vi "Main.vi"(11 "Module Admin":refnum<class "Delacor_lib_QMH_Module Admin.lvclass">) -> ()   [LabVIEW 2020, in "Hardware.lvlib"]
doc: "This template is based off of the Queued Message Handler design pattern and the Queued Message Handler project template that ships with LabVIEW.\n\nThe main difference is that the queue is private to this module and communication between modules is performed via Broadcast and Request events.\n\nRequest events are wrapped in public API methods and are handled in the Event Handling Loop (EHL) of this VI. Any module can register for Broadcast events sent by this module. The EHL generates messages based on user interface actions.\n\nThe Message Handling Loop (MHL) processes messages generated by the EHL, or by other messages. The messages are string values, so new messages can be added easily to the Message Cases case structure in the MHL. Each message cluster can also provide an optional value for Message Data, which is a variant that can be converted to whatever message-specific data is required.\n_____\nBased on DQMH Project Template 6.0.0.91."
uses:
  Hardware.lvlib
  <vilib>/Delacor/Delacor QMH/Libraries/Module Admin_class/Delacor_lib_QMH_Module Admin.lvclass
  Module Data--cluster.ctl
  Stop Argument--cluster.ctl
  <vilib>/Delacor/Delacor QMH/Libraries/Message Queue_class/Delacor_lib_QMH_Message Queue.lvclass/Delacor_lib_QMH_Message Queue.ctl
  <vilib>/Delacor/Delacor QMH/Libraries/Module Admin_class/Delacor_lib_QMH_Module Admin.lvclass/Delacor_lib_QMH_Module Admin.ctl
  <vilib>/Utility/miscctls.llb/LVPointTypeDef.ctl
  <vilib>/Delacor/Delacor QMH/Libraries/Message Queue_class/Delacor_lib_QMH_Enqueue Message (Single).vi
  <vilib>/Delacor/Delacor QMH/Libraries/Module Admin_class/Delacor_lib_QMH_Get External Launch.vi
  <vilib>/Utility/error.llb/Error Cluster From Error Code.vi
  <vilib>/ErrorRing/Error Ring.xnode
  <vilib>/Delacor/Delacor QMH/Libraries/Message Queue_class/Delacor_lib_QMH_Message Queue.lvclass
  Paquetes Disponibles/Paquetes Disponibles.lvlib
  Manejador Turnos/Manejador Turnos.lvlib
panel:
  out "error out":errorcluster
  out "Status":string
types:
  T1 = typedef "Hardware.lvlib/Request Events--cluster.ctl" = cluster{"Stop Module":refnum<user-event>, "Show Panel":refnum<user-event>, "Hide Panel":refnum<user-event>, "Get Module Execution Status":refnum<user-event>, "Show Diagram":refnum<user-event>}
  T2 = typedef "Manejador Turnos.lvlib/Broadcast Events--cluster.ctl" = cluster{"Module Did Init":refnum<user-event>, "Status Updated":refnum<user-event>, "Error Reported":refnum<user-event>, "Module Did Stop":refnum<user-event>, "Update Module Execution Status":refnum<user-event>, "Servicio en curso":refnum<user-event>}
  T3 = typedef "Hardware.lvlib/Module Data--cluster.ctl" = cluster{"Status":string, "Servicio":string}
  T4 = enum32{"invalid lock state", "Not Locked", "Locked (No Password)", "Password-protected"}
  T5 = typedef "Hardware.lvlib/Stop Argument--cluster.ctl" = cluster{"Origin":string, "Exit via Stop Module Req?":bool, "Wait for Module to stop?":bool}
  T6 = typedef "LVPointTypeDef.ctl" = cluster{"Horizontal":i16, "Vertical":i16}
  T7 = enum32{"Invalid", "Standard", "Closed", "Hidden", "Minimized", "Maximized"}
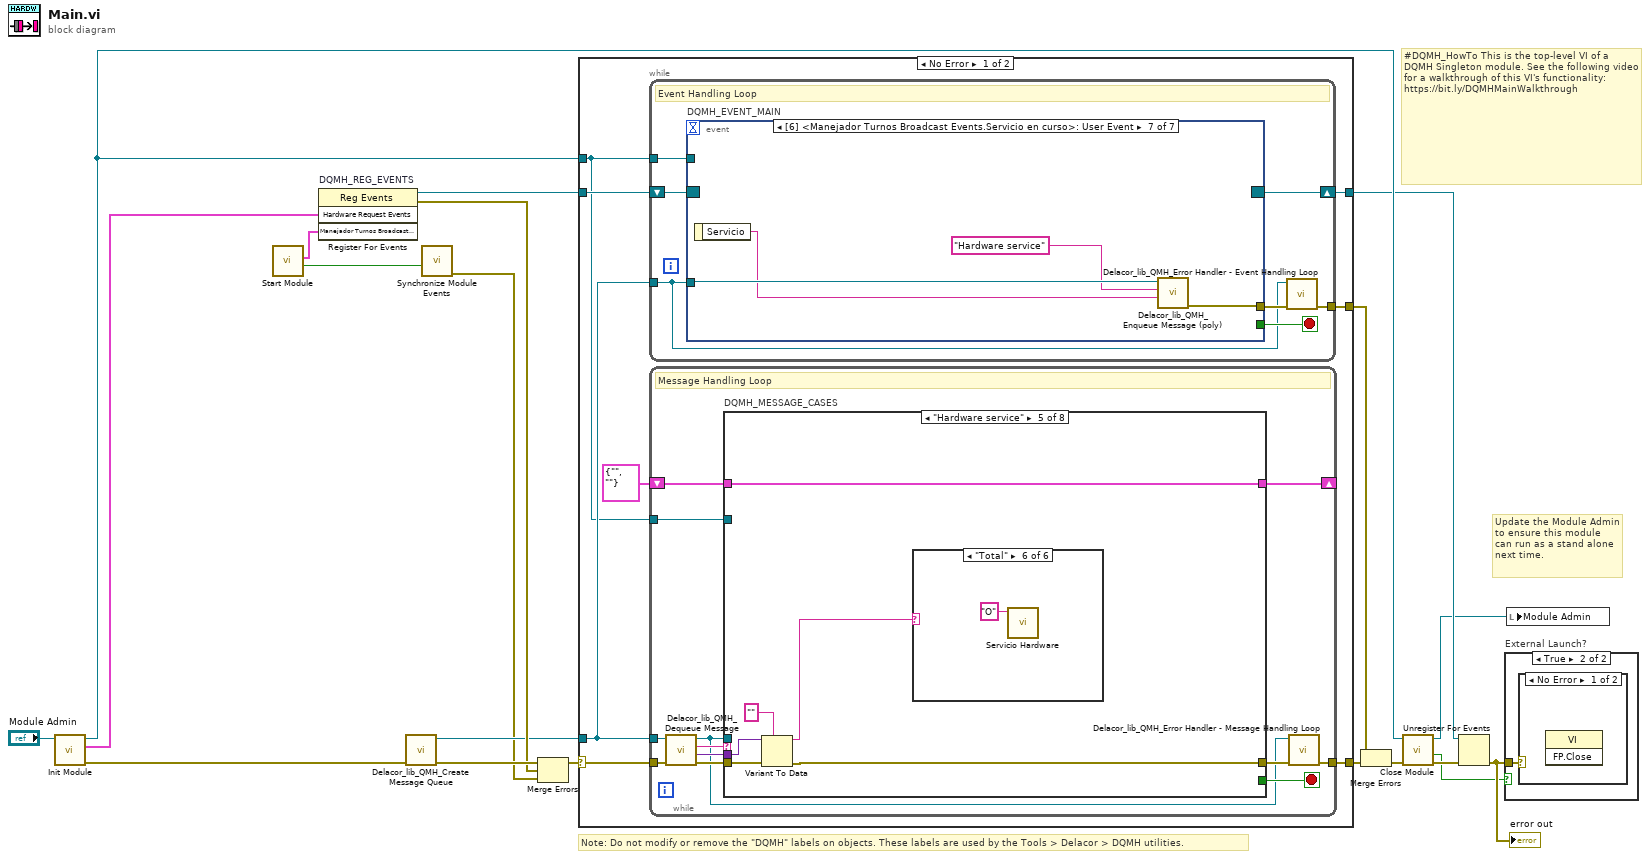
[diagram p0: block diagram]
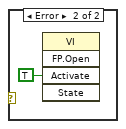
[diagram p3: hidden frame]
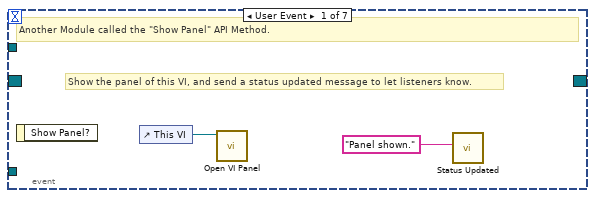
[diagram p4: hidden frame]
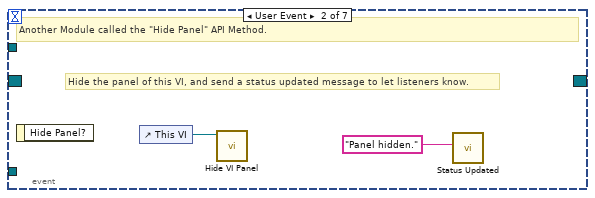
[diagram p5: hidden frame]
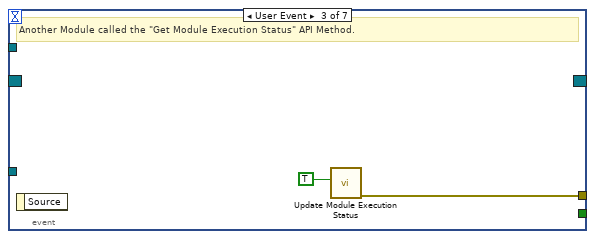
[diagram p6: hidden frame]
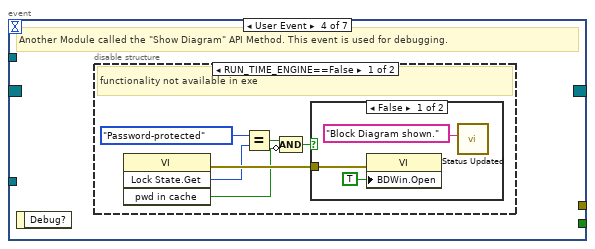
[diagram p7: hidden frame]
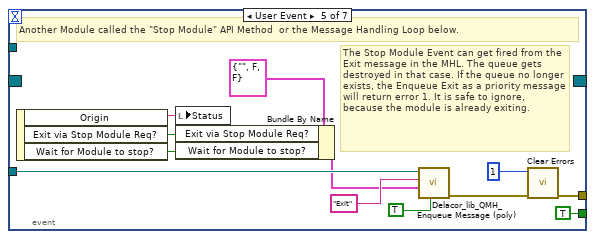
[diagram p10: hidden frame]
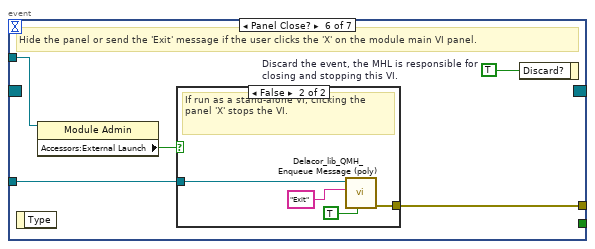
[diagram p11: hidden frame]
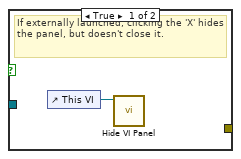
[diagram p12: hidden frame]
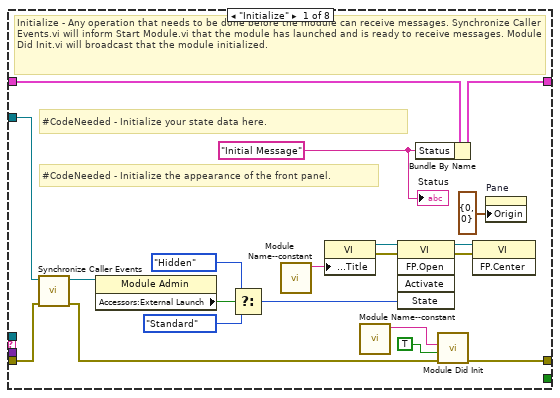
[diagram p13: hidden frame]
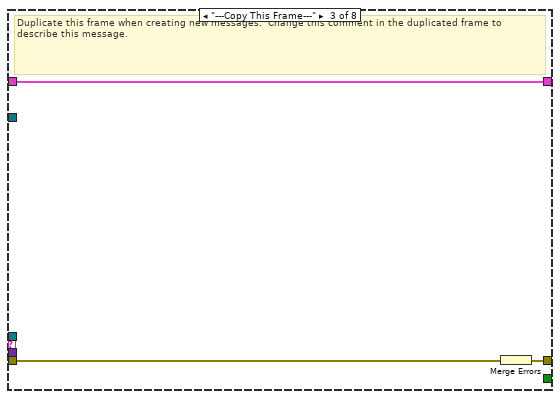
[diagram p15: hidden frame]
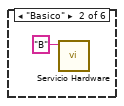
[diagram p18: hidden frame]
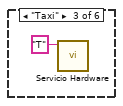
[diagram p19: hidden frame]
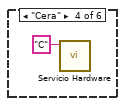
[diagram p20: hidden frame]
diagram:
  # "#DQMH_HowTo This is the top-level VI of a DQMH Singleton module. See the following video for a walkthrough of this VI's functionality: https://bit.ly/DQMHMainWalkthrough"
  # "Note: Do not modify or remove the \"DQMH\" labels on objects. These labels are used by the Tools > Delacor > DQMH utilities."
  # "Update the Module Admin to ensure this module can run as a stand alone next time."
  n1 = call "Init Module.vi"("Singleton Module Admin in"="Module Admin") -> ("error out"=w19:errorcluster, "Hardware Request Events"=w8:T1, "Singleton Module Admin out"=w11:refnum<class "Delacor_lib_QMH_Module Admin.lvclass">)  [unwired: 8 in]
  n2 = call "Start Module.vi"() -> ("Wait for Event Sync?"=w3:bool, "Manejador Turnos Broadcast Events"=w1:T2)  [unwired: 8 in, 2 out]
  n3 = register-events "DQMH_REG_EVENTS"(w8, w1) -> (reference out=w9:refnum<event-registration>, error out=w12:errorcluster)  [unwired: 2 in]
  n4 = call <vilib>:"Delacor_lib_QMH_Create Message Queue.vi"("error in"=w19) -> ("error out"=w14:errorcluster, "Message Queue"=w7:refnum<class "Delacor_lib_QMH_Message Queue.lvclass">)  [unwired: 9 in]
  n5 = call "Synchronize Module Events.vi"("Wait for Event Sync?"=w3) -> ("error out"=w2:errorcluster)  [unwired: 10 in]
  n6 = Merge Errors(w14, w12, w2) -> (w13:errorcluster)
  n7 = case shown="No Error" w13 {
    selector: w13 -> [w26 w174]
    tunnel: [w28 w173] -> w20
    tunnel: [w25 w179] -> w10
    tunnel: w9 -> [w23 w179]
    tunnel: w7 -> [w22 w172]
    tunnel: [w27 _] -> w17
    tunnel: w11 -> [w21 w175]
    frame No Error {
      n8 = while {
        tunnel: w22 -> [w29]
        shift-right: [w32] -> w25
        shift-left: w23 -> [w33]
        tunnel: [w34] -> w27
        tunnel: w21 -> [w30]
        stop <- w31 stop-if-true
        # "Event Handling Loop"
        n9 = event "DQMH_EVENT_MAIN" shown="[6] <Manejador Turnos Broadcast Events.Servicio en curso>: User Event" {
          selector: w33 -> [_ _ _ _ _ _ _]
          dyn-events: [_ _ _ _ _ _ _] -> w32
          timeout: _ -> [_ _ _ _ _ _ _]
          tunnel: [_ _ _ _ TRUE ("Discard?") _ _] -> w31
          tunnel: w29 -> [_ _ _ _ w58 w65 w75]
          tunnel: [_ _ w41 _ w61 w67 w76] -> w35
          tunnel: w30 -> [_ _ _ _ _ w64 _]
          event User Event {
            # "Show the panel of this VI, and send a status updated message to let listeners know."
            # "Another Module called the \"Show Panel\" API Method."
            n10 = event-data() -> ()  [unwired: 1 in, 1 out]
            n11 = control-ref of="This VI"() -> (w37:refnum<vi>)
            n12 = call "Open VI Panel.vi"("VI"=w37) -> ()  [unwired: 10 in, 1 out]
            n13 = call "Status Updated.vi"("Status"="Panel shown." ("format string")) -> ()  [unwired: 10 in, 1 out]
          }
          event User Event {
            # "Hide the panel of this VI, and send a status updated message to let listeners know."
            # "Another Module called the \"Hide Panel\" API Method."
            n14 = event-data() -> ()  [unwired: 1 in, 1 out]
            n15 = control-ref of="This VI"() -> (w39:refnum<vi>)
            n16 = call "Hide VI Panel.vi"("VI"=w39) -> ()  [unwired: 10 in, 1 out]
            n17 = call "Status Updated.vi"("Status"="Panel hidden." ("format string")) -> ()  [unwired: 10 in, 1 out]
          }
          event User Event {
            # "Another Module called the \"Get Module Execution Status\" API Method."
            n18 = event-data() -> ()  [unwired: 1 in, 1 out]
            n19 = call "Update Module Execution Status.vi"("Running?"=TRUE) -> ("error out"=w41:errorcluster)  [unwired: 10 in]
          }
          event User Event {
            # "Another Module called the \"Show Diagram\" API Method. This event is used for debugging."
            n20 = event-data() -> ()  [unwired: 1 in, 1 out]
            n21 = disable-structure shown="RUN_TIME_ENGINE==False" {
              frame condition #0 (active) {
                # "functionality not available in exe"
                n22 = invoke class="VI" method="Lock State.Get"() -> (error out=w47:errorcluster, "Get Lock State"=w46:T4, "pwd in cache"=w43:bool)  [unwired: 4 in, 1 out]
                n23 = Equal?(x=T4."Password-protected", y=w46) -> (x = y?=w44:bool)
                n24 = Compound Arithmetic op=AND(w44, invert w43) -> (w42:bool)
                n25 = case shown="False" w42 {
                  tunnel: w47 -> [w50 _]
                  frame False {
                    n26 = property class="VI"(error in=w50, "BDWin.Open"=TRUE ("Block Diagram Window:Open")) -> ()  [unwired: 1 in, 2 out]
                    n27 = call "Status Updated.vi"("Status"="Block Diagram shown." ("format string")) -> ()  [unwired: 10 in, 1 out]
                  }
                  frame True {
                    # "Password-protected VI, and the password is not in the cache. Do not show the diagram."
                  }
                }
              }
              frame condition #1 {
              }
            }
          }
          event User Event {
            # "The Stop Module Event can get fired from the Exit message in the MHL. The queue gets destroyed in that case. If the queue no longer exists, the Enqueue Exit as a priority message will return error 1. It is safe to ignore, because the module is already exiting."
            # "Another Module called the \"Stop Module\" API Method  or the Message Handling Loop below."
            n28 = event-data() -> ("Origin"=w57:string, "Exit via Stop Module Req?"=w53:bool, "Wait for Module to stop?"=w52:bool)  [unwired: 1 in]
            n29 = local write "Status"(w57) -> ()
            n30 = Bundle By Name(cluster=T5 {"Origin"="", "Exit via Stop Module Req?"=FALSE, "Wait for Module to stop?"=FALSE} ("Stop Argument"), "Exit via Stop Module Req?"=w53, "Wait for Module to stop?"=w52) -> (w51:T5)
            n31 = call-poly <vilib>:"Delacor_lib_QMH_Enqueue Message (poly).vi"("Priority Message? (F)"=TRUE, "Message Data"=w51, "Message"="Exit", "Message Queue in"=w58) -> ("error out"=w62:errorcluster)  [unwired: 6 in, 1 out]
            n32 = call <vilib>:"Clear Errors.vi"("error in (no error)"=w62, "specific error code to clear (0: all)"=1) -> ("error out"=w61:errorcluster)  [unwired: 4 in, 1 out]
          }
          event Panel Close? {
            w66 = TRUE  # Discard the event, the MHL is responsible for closing and stopping this VI.
            # "Hide the panel or send the 'Exit' message if the user clicks the 'X' on the module main VI panel."
            n33 = event-data() -> ()  [unwired: 1 in, 1 out]
            n34 = property class="Module Admin"(reference=w64) -> ("Accessors:External Launch"=w63:bool)  [unwired: 1 in, 2 out]
            n35 = case shown="False" w63 {
              tunnel: w65 -> [_ w71]
              tunnel: [_ w72] -> w67
              frame True {
                # "If externally launched, clicking the 'X' hides the panel, but doesn't close it."
                n36 = control-ref of="This VI"() -> (w68:refnum<vi>)
                n37 = call "Hide VI Panel.vi"("VI"=w68) -> ()  [unwired: 10 in, 1 out]
              }
              frame False {
                # "If run as a stand-alone VI, clicking the panel 'X' stops the VI."
                n38 = call-poly <vilib>:"Delacor_lib_QMH_Enqueue Message (poly).vi"("Priority Message? (F)"=TRUE, "Message"="Exit", "Message Queue in"=w71) -> ("error out"=w72:errorcluster)  [unwired: 7 in, 1 out]
              }
            }
            n39 = event-data("Discard?"=w66) -> ()  [unwired: 1 in, 1 out]
          }
          event User Event {
            n40 = event-data() -> ("Servicio"=w74:string)  [unwired: 1 in]
            n41 = call-poly <vilib>:"Delacor_lib_QMH_Enqueue Message (poly).vi"("Message Data"=w74, "Message"="Hardware service", "Message Queue in"=w75) -> ("error out"=w76:errorcluster)  [unwired: 7 in, 1 out]
          }
        }
        n42 = call-dynamic "Delacor_lib_QMH_Error Handler - Event Handling Loop.vi"("error in"=w35, "Message Queue in"=w29) -> ("dup error in"=w34:errorcluster)  [unwired: 8 in, 1 out]
      }
      n43 = while {
        tunnel: w22 -> [w79]
        shift-right: [w83] -> _
        shift-left: T3 {"Status"="", "Servicio"=""} ("Data Cluster") -> [w84]
        tunnel: w26 -> [w87]
        tunnel: [w85] -> w28
        tunnel: w21 -> [w77]
        stop <- w82 stop-if-true
        # "Message Handling Loop"
        n44 = call-dynamic "Delacor_lib_QMH_Dequeue Message.vi"("error in"=w87, "Message Queue in"=w79) -> ("error out"=w86:errorcluster, "Message Data"=w80:variant, "Message"=w81:string, "Message Queue out"=w78:refnum<class "Delacor_lib_QMH_Message Queue.lvclass">)  [unwired: 6 in]
        n45 = case "DQMH_MESSAGE_CASES" shown="\"Hardware service\"" w81 {
          selector: w81 -> [_ _ _ _ _ _ _ w159]
          tunnel: w78 -> [_ _ _ _ _ w129 w151 _]
          tunnel: w86 -> [w106 w110 w113 w115 w120 w136 w157 w161]
          tunnel: [w104 w110 w112 w115 w118 w132 w154 w162] -> w88
          tunnel: w84 -> [w95 w109 w111 w114 w121 w131 w150 w160]
          tunnel: [w94 w109 w111 w114 w121 w131 w150 w160] -> w83
          tunnel: [_ _ _ _ _ _ w149 _] -> w82
          tunnel: w80 -> [_ _ _ _ w119 w130 w148 _]
          tunnel: w77 -> [w96 _ _ _ _ w128 w143 _]
          frame "Initialize" {
            w90 = "Initial Message" ("Initial Message")
            # "#CodeNeeded - Initialize the appearance of the front panel."
            # "#CodeNeeded - Initialize your state data here."
            # "Initialize - Any operation that needs to be done before the module can receive messages. Synchronize Caller Events.vi will inform Start Module.vi that the module has launched and is ready to receive messages. Module Did Init.vi will broadcast that the module initialized."
            n46 = call "Synchronize Caller Events.vi"("error in (no error)"=w106, "Singleton Module Admin in"=w96) -> ("error out"=w105:errorcluster, "Singleton Module Admin out"=w91:refnum<class "Delacor_lib_QMH_Module Admin.lvclass">)  [unwired: 8 in]
            n47 = property class="Module Admin"(reference=w91) -> ("Accessors:External Launch"=w100:bool)  [unwired: 1 in, 2 out]
            n48 = Select(t=T7."Hidden" ("State"), s=w100, f=T7."Standard" ("State")) -> (s? t:f=w97:T7)
            n49 = call "Module Name--constant.vi"() -> ("Module Name"=w103:string)  [unwired: 11 in]
            n50 = property class="VI"("Front Panel.Title"=w103) -> (reference out=w102:refnum<vi>, error out=w108:errorcluster)  [unwired: 2 in]
            n51 = call "Module Name--constant.vi"() -> ("Module Name"=w92:string)  [unwired: 11 in]
            n52 = invoke class="VI" method="FP.Open"(reference=w102, error in=w108, "State"=w97) -> (reference out=w101:refnum<vi>, error out=w107:errorcluster)  [unwired: 2 in, 3 out]
            n53 = Bundle By Name(cluster=w95, "Status"=w90) -> (w94:T3)
            n54 = call "Module Did Init.vi"("error in (no error)"=w105, "Initialized?"=TRUE, "Origin"=w92) -> ("error out"=w104:errorcluster)  [unwired: 8 in]
            n55 = invoke class="VI" method="FP.Center"(reference=w101, error in=w107) -> ()  [unwired: 1 in, 3 out]
            n56 = property on="Pane" class="Pane"("Origin"=T6 {"Horizontal"=0, "Vertical"=0}) -> ()  [unwired: 2 in, 2 out]
            "Status" <- w90
          }
          frame "---Module Specific---" {
            # "Separator -- The following cases handle messages specific to this Module."
          }
          frame "---Copy This Frame---" {
            # "Duplicate this frame when creating new messages.  Change this comment in the duplicated frame to describe this message."
            n57 = Merge Errors(w113) -> (w112:errorcluster)
          }
          frame "---Exit and Error Handling---" {
            # "Separator - The following cases handle errors and exit messages."
          }
          frame "Hardware service" {
            n58 = Variant To Data(error in=w120, type="", Variant=w119) -> (data=w116:string, error out=w118:errorcluster)
            n59 = case shown="\"Total\"" w116 {
              frame Default {
              }
              frame "Basico" {
                n60 = call "Servicio Hardware.vi"("Caracter Servicio"="B") -> ()  [unwired: 10 in, 1 out]
              }
              frame "Taxi" {
                n61 = call "Servicio Hardware.vi"("Caracter Servicio"="T") -> ()  [unwired: 10 in, 1 out]
              }
              frame "Cera" {
                n62 = call "Servicio Hardware.vi"("Caracter Servicio"="C") -> ()  [unwired: 10 in, 1 out]
              }
              frame "Motor" {
                n63 = call "Servicio Hardware.vi"("Caracter Servicio"="M") -> ()  [unwired: 10 in, 1 out]
              }
              frame "Total" {
                n64 = call "Servicio Hardware.vi"("Caracter Servicio"="O") -> ()  [unwired: 10 in, 1 out]
              }
            }
          }
          frame "Error" {
            # "#CodeRecommended - If you ever change the name of this \"Error\" message, you'll need to update the name in the Check Loop Error.vi as well."
            # "#CodeRecommended - If the module is running in standalone mode (External Launch = FALSE), this code will pop up an error dialog and call the 'Exit' message if an error occurs. Add more fine-grained error handling here."
            # "Error - Check the error message data and respond accordingly. This message is sent by the \"Error Handler\" VIs at the end of each loop in this application."
            n65 = property class="Module Admin"(reference=w128) -> ("Accessors:External Launch"=w127:bool)  [unwired: 1 in, 2 out]
            n66 = Variant To Data(error in=w136, type=errorcluster {"status"=FALSE, "code"=0, "source"=""} ("error constant"), Variant=w130) -> (data=w137:errorcluster, error out=w134:errorcluster)
            n67 = call "Error Reported.vi"("Error"=w137) -> ()  [unwired: 10 in, 1 out]
            n68 = case shown="False" w127 {
              tunnel: [w142 _] -> w133
              tunnel: w129 -> [w140 _]
              tunnel: w137 -> [w141 _]
              frame False {
                # "If the module is running standalone, then pop up an error dialog and call the \"Exit\" message."
                n69 = call <vilib>:"Simple Error Handler.vi"("error in (no error)"=w141) -> ()  [unwired: 4 in, 5 out]
                n70 = call-poly <vilib>:"Delacor_lib_QMH_Enqueue Message (poly).vi"("Priority Message? (F)"=TRUE, "Message"="Exit", "Message Queue in"=w140) -> ("error out"=w142:errorcluster)  [unwired: 7 in, 1 out]
              }
              frame True {
                # "If the module was launched externally, calling the Error Reported broadcast VI is the only action performed by the \"Error\" message. The module's caller can then process the error appropriately."
              }
            }
            n71 = Merge Errors(w134, w133) -> (w132:errorcluster)
            n72 = local write "error out"(w132) -> ()
          }
          frame "Exit" {
            w147 = 91  # 91: not all Exit messages will have an argument
            w149 = TRUE  # Stop the VI
            # "Release the message queue reference"
            # "#CodeNeeded - Add any required cleanup code here"
            # "Exit - Exit the application."
            n73 = Variant To Data(error in=w157, type=T5 {"Origin"="", "Exit via Stop Module Req?"=FALSE, "Wait for Module to stop?"=FALSE} ("Stop Argument"), Variant=w148) -> (data=w145:T5, error out=w153:errorcluster)
            n74 = call <vilib>:"Clear Errors.vi"("error in (no error)"=w153, "specific error code to clear (0: all)"=w147) -> ("error out"=w156:errorcluster)  [unwired: 4 in, 1 out]
            n75 = control-ref of="This VI"() -> (w144:refnum<vi>)
            n76 = call-dynamic "Delacor_lib_QMH_Release Message Queue.vi"("error in"=w156, "Message Queue"=w151) -> ("error out"=w155:errorcluster)  [unwired: 9 in]
            n77 = call "Handle Exit.vi"("Stop Argument"=w145, "Admin in"=w143, "VI reference"=w144) -> ("error out"=w152:errorcluster)  [unwired: 7 in, 1 out]
            n78 = Merge Errors(w155, w152) -> (w154:errorcluster)
            n79 = call "Stop Module.vi"() -> ()  [unwired: 11 in, 1 out]
          }
          frame Default {
            # "'Default' case only runs if there is a message that isn't defined in any of the other cases.  Output a programming error."
            n80 = call "Module Name--constant.vi"() -> ("Module Name"=w158:string)  [unwired: 11 in]
            n81 = xnode "Error Ring"("parameter 0"=w159, "parameter 1"=w158) -> ("error out"=w163:errorcluster)
            n82 = Merge Errors(w161, w163) -> (w162:errorcluster)
          }
        }
        n83 = call-dynamic "Delacor_lib_QMH_Error Handler - Message Handling Loop.vi"("error in"=w88, "Message Queue in"=w78) -> ("dup error in"=w85:errorcluster)  [unwired: 8 in, 1 out]
      }
    }
    frame Error {
      # "Synchronize Caller Events.vi will inform Start Module.vi that the module has launched and will let the code calling Start Module.vi register for broadcasts and would permit the caller receive the broadcast that an error occurred at launch time."
      n84 = call-dynamic "Delacor_lib_QMH_Release Message Queue.vi"("error in"=w174, "Message Queue"=w172) -> ("error out"=w173:errorcluster)  [unwired: 9 in]
      n85 = call "Synchronize Caller Events.vi"("Singleton Module Admin in"=w175) -> ("error out"=w180:errorcluster)  [unwired: 9 in, 1 out]
      n86 = call "Module Name--constant.vi"() -> ("Module Name"=w178:string)  [unwired: 11 in]
      n87 = Format Into String(format string="An error occurred during initialization. %s is no longer running.", w178) -> (resulting string=w176:string)  [unwired: 2 in, 1 out]
      n88 = Merge Errors(w173, w180) -> (w181:errorcluster)
      n89 = call "Stop Module.vi"() -> ()  [unwired: 11 in, 1 out]
      n90 = call "Error Reported.vi"("Additional Information"=w176, "Error"=w181) -> ()  [unwired: 9 in, 1 out]
      n91 = call "Stop Module.vi"() -> ()  [unwired: 11 in, 1 out]
    }
  }
  n92 = Merge Errors(w17, w20) -> (w16:errorcluster)
  n93 = call "Close Module.vi"("error in (no error)"=w16, "Module Admin in"=w11) -> ("error out"=w18:errorcluster, "External Launch"=w4:bool, "Module Admin out"=w5:refnum<class "Delacor_lib_QMH_Module Admin.lvclass">)  [unwired: 7 in]
  n94 = Unregister For Events(event registration refnum=w10, error in=w18) -> (error out=w15:errorcluster)
  "error out" <- w15
  n95 = case "External Launch?" shown="True" w4 {
    tunnel: w15 -> [_ w182]
    frame False {
    }
    frame True {
      n96 = case shown="No Error" w182 {
        frame No Error {
          n97 = invoke class="VI" method="FP.Close"() -> ()  [unwired: 3 in, 3 out]
        }
        frame Error {
          n98 = invoke class="VI" method="FP.Open"("Activate"=TRUE ("Activate?")) -> ()  [unwired: 4 in, 5 out]
        }
      }
    }
  }
  n99 = local write "Module Admin"(w5) -> ()
